vi "Init Draw Characters.vi"(8 "error in (no error)":errorcluster, 10 "Characters Initial Pos":T1[](array[typedef]), 11 "Draw in":refnum<class "Draw.lvclass">) -> (0 "error out":errorcluster, 3 "Draw out":refnum<class "Draw.lvclass">)   [LabVIEW 2016, in "PacManClasses.lvlib" / "Draw.lvclass"]
uses:
  Draw.lvclass
  Generic Controls/Point.ctl
  Circle/PacMan.lvclass
  C:/Users/lucamach/Documents/SE/Learning OOP/PacMan/PacMan Classes/Geometric Figure/UI Object.lvclass
  Generic Controls/Picture.ctl
  Generic Controls/Color.ctl
  Generic Controls/Pen.ctl
  Generic Controls/Size - Bounding Rect.ctl
  Generic Controls/Ghosts.ctl
  Geometric Figure/UI Object.lvclass/UI Object.ctl
  Character/Ghosts.lvclass
  Geometric Figure/Write Center (px).vi
  Geometric Figure/Write Color (RGB).vi
  PacManClasses.lvlib
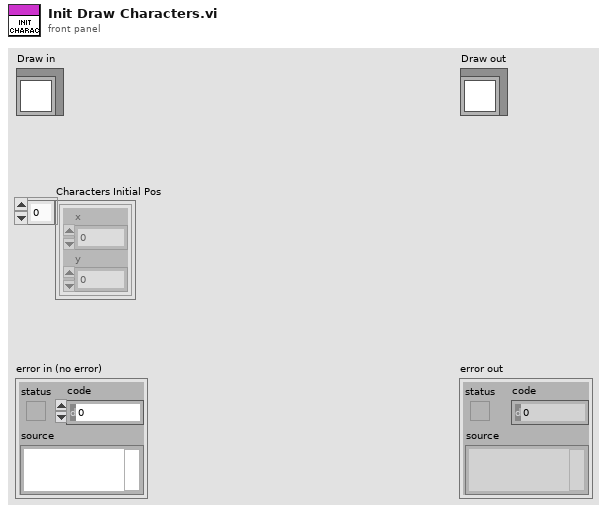
[diagram p1: front panel]
types:
  T1 = typedef "PacManClasses.lvlib/Point.ctl" = cluster{"x":u16, "y":u16}
  T2 = typedef "PacManClasses.lvlib/Size - Bounding Rect.ctl" = cluster{"Width":u16, "Height":u16}
  T3 = typedef "PacManClasses.lvlib/Pen.ctl" = cluster{"Width":u16, "Style":enum32{"Solid", "Dash", "Dot", "DashDot", "DashDotDot"}}
  T4 = typedef "PacManClasses.lvlib/Color.ctl" = cluster{"Red":u8, "Green":u8, "Blue":u8}
  T5 = typedef "PacManClasses.lvlib/Ghosts.ctl" = enum16{"Blinky", "Pinky", "Inky", "Clyde"}
  T6 = typedef "PacManClasses.lvlib/Picture.ctl" = picture
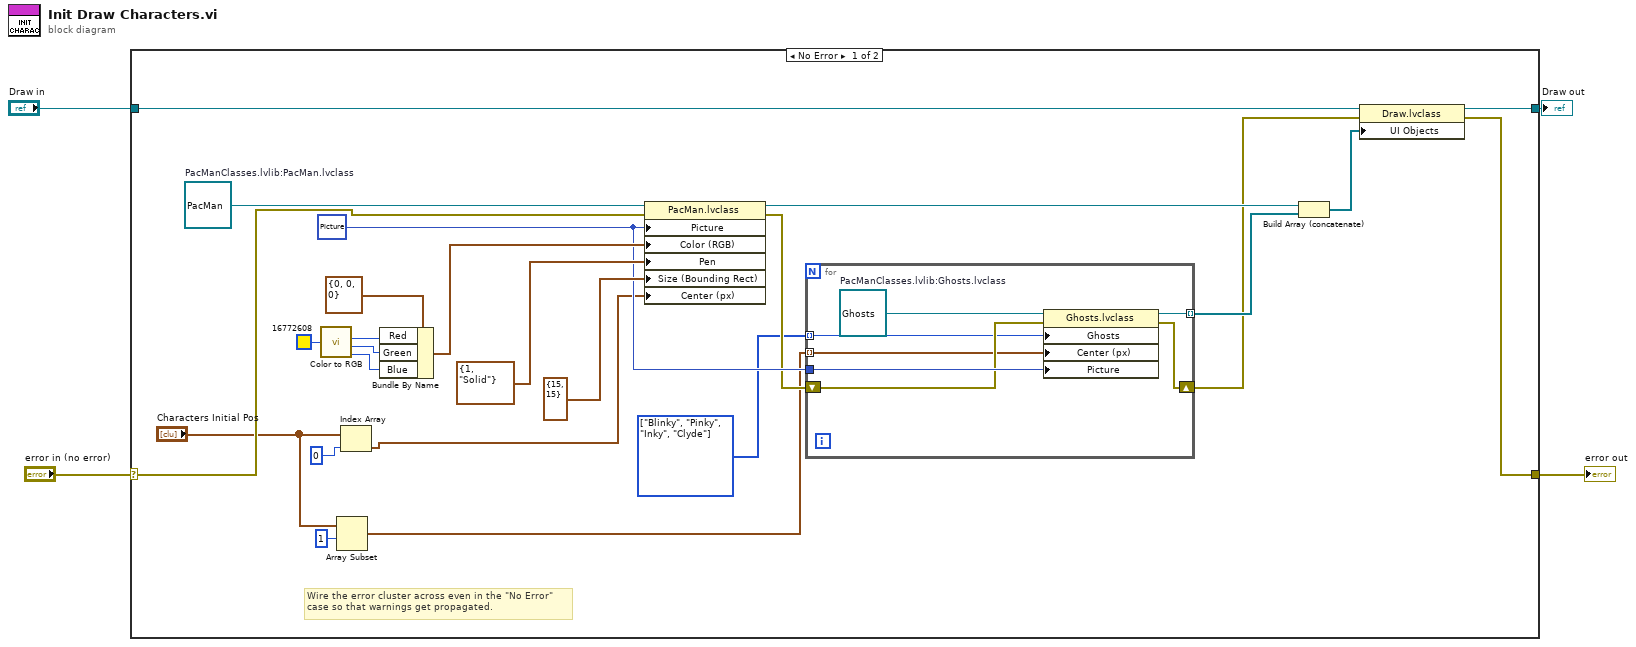
[diagram p0: block diagram]
diagram:
  n1 = case shown="No Error" "error in (no error)" {
    selector: "error in (no error)" -> [w7 w38]
    tunnel: [w6 w38] -> w3
    tunnel: [w8 w37] -> w1
    tunnel: "Draw in" -> [w9 w37]
    frame No Error {
      w15 = T5[] [enum."Blinky", enum."Pinky", enum."Inky", enum."Clyde"] items=["Blinky", "Pinky", "Inky", "Clyde"]
      w18 = T6 data[5B] ("Picture")
      w27 = refnum<class "PacMan.lvclass"> refnum  # PacManClasses.lvlib:PacMan.lvclass
      # "Wire the error cluster across even in the \"No Error\"\ncase so that warnings get propagated."
      n2 = call <vilib>:"Color to RGB.vi"("Color"=u32 16772608) -> ("R"=w23:u8, "G"=w24:u8, "B"=w25:u8)  [unwired: 1 out]
      n3 = Array Subset(array="Characters Initial Pos", index=1) -> (w10:T1[])  [unwired: 1 in]
      n4 = Index Array(array="Characters Initial Pos", index=0 ("length")) -> (element=w12:T1)
      n5 = Bundle By Name(cluster=T4 {"Red"=0, "Green"=0, "Blue"=0} ("Color (RGB)"), "Red"=w23, "Green"=w24, "Blue"=w25) -> (w28:T4)
      n6 = property class="PacMan.lvclass"(reference=w27, error in=w7, "Picture"=w18, "Color (RGB)"=w28, "Pen"=T3 {"Width"=1, "Style"=enum."Solid"} ("pen"), "Size (Bounding Rect)"=T2 {"Width"=15, "Height"=15}, "Center (px)"=w12) -> (reference out=w21:refnum<class "PacMan.lvclass">, error out=w17:errorcluster)
      n7 = for {
        tunnel: w18 -> [w36]
        shift-right: [w34] -> w14
        shift-left: w17 -> [w35]
        tunnel: [w32] -> w16 mode=indexing
        tunnel: w15 -> [w31] mode=indexing
        tunnel: w10 -> [w30] mode=indexing
        w33 = refnum<class "Ghosts.lvclass"> refnum  # PacManClasses.lvlib:Ghosts.lvclass
        n8 = property class="Ghosts.lvclass"(reference=w33, error in=w35, "Ghosts"=w31, "Center (px)"=w30, "Picture"=w36) -> (reference out=w32:refnum<class "Ghosts.lvclass">, error out=w34:errorcluster)
      }
      n9 = Build Array (concatenate)(w21, w16) -> (w20:refnum<class "UI Object.lvclass">[])
      n10 = property class="Draw.lvclass"(reference=w9, error in=w14, "UI Objects"=w20) -> (reference out=w8:refnum<class "Draw.lvclass">, error out=w6:errorcluster)
    }
    frame Error {
    }
  }
  "error out" <- w3
  "Draw out" <- w1
